vi "SetMDT69Value.vi"(8 "error in (no error)":errorcluster, 9 "Value":string, 10 "Channel":string, 11 "VISA resource name":refnum<visa-resource-name>) -> (0 "error out":errorcluster, 3 "VISA resource name":refnum<visa-resource-name>)   [LabVIEW 2020]
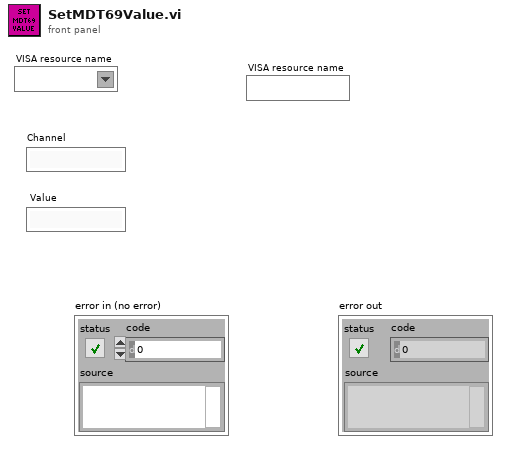
[diagram p1: front panel]
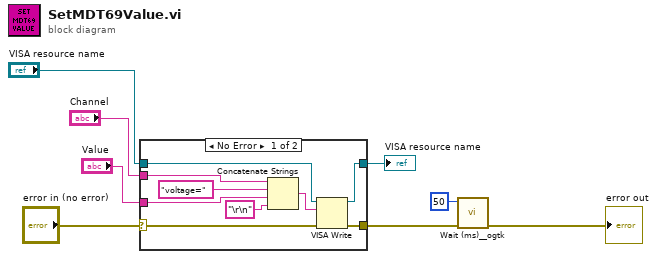
[diagram p0: block diagram]
diagram:
  n1 = case shown="No Error" "error in (no error)" {
    selector: "error in (no error)" -> [w11 w19]
    tunnel: [w10 w19] -> w3
    tunnel: "VISA resource name" -> [w13 w18]
    tunnel: [w12 w18] -> w6
    tunnel: "Channel" -> [w17 _]
    tunnel: "Value" -> [w15 _]
    frame No Error {
      n2 = Concatenate Strings(w17, "voltage=" ("string"), w15, "\r\n" ("string")) -> (w14:string)
      n3 = VISA Write(VISA resource name=w13, write buffer=w14, error in (no error)=w11) -> (VISA resource name out=w12:refnum<visa-resource-name>, error out=w10:errorcluster)  [unwired: 1 out]
    }
    frame Error {
    }
  }
  "VISA resource name" <- w6
  n4 = call "Wait (ms)__ogtk.vi"("error in (no error)"=w3, "milliseconds to wait"=u32 50) -> ("error out"=→"error out":errorcluster)  [unwired: 8 in, 1 out]
